vi "Wind Blowing Blizzards.vi"(1 "Valley in":T1[][](array[typedef])) -> (0 "Valley out":T1[][](array[typedef]))   [LabVIEW 2020, in "AoC 2022.lvlib"]
uses:
  AoC 2022.lvlib
  Valley Point.ctl
  Valley Item.ctl
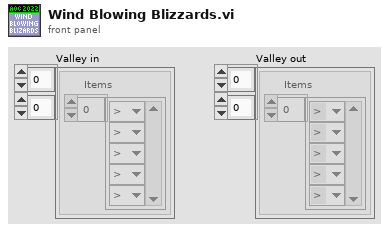
[diagram p1: front panel]
types:
  T1 = typedef "AoC 2022.lvlib/Valley Point.ctl" = cluster{"Items":T2[]}
  T2 = typedef "AoC 2022.lvlib/Valley Item.ctl" = enum16{"#", ".", ">", "<", "^", "v", "E"}
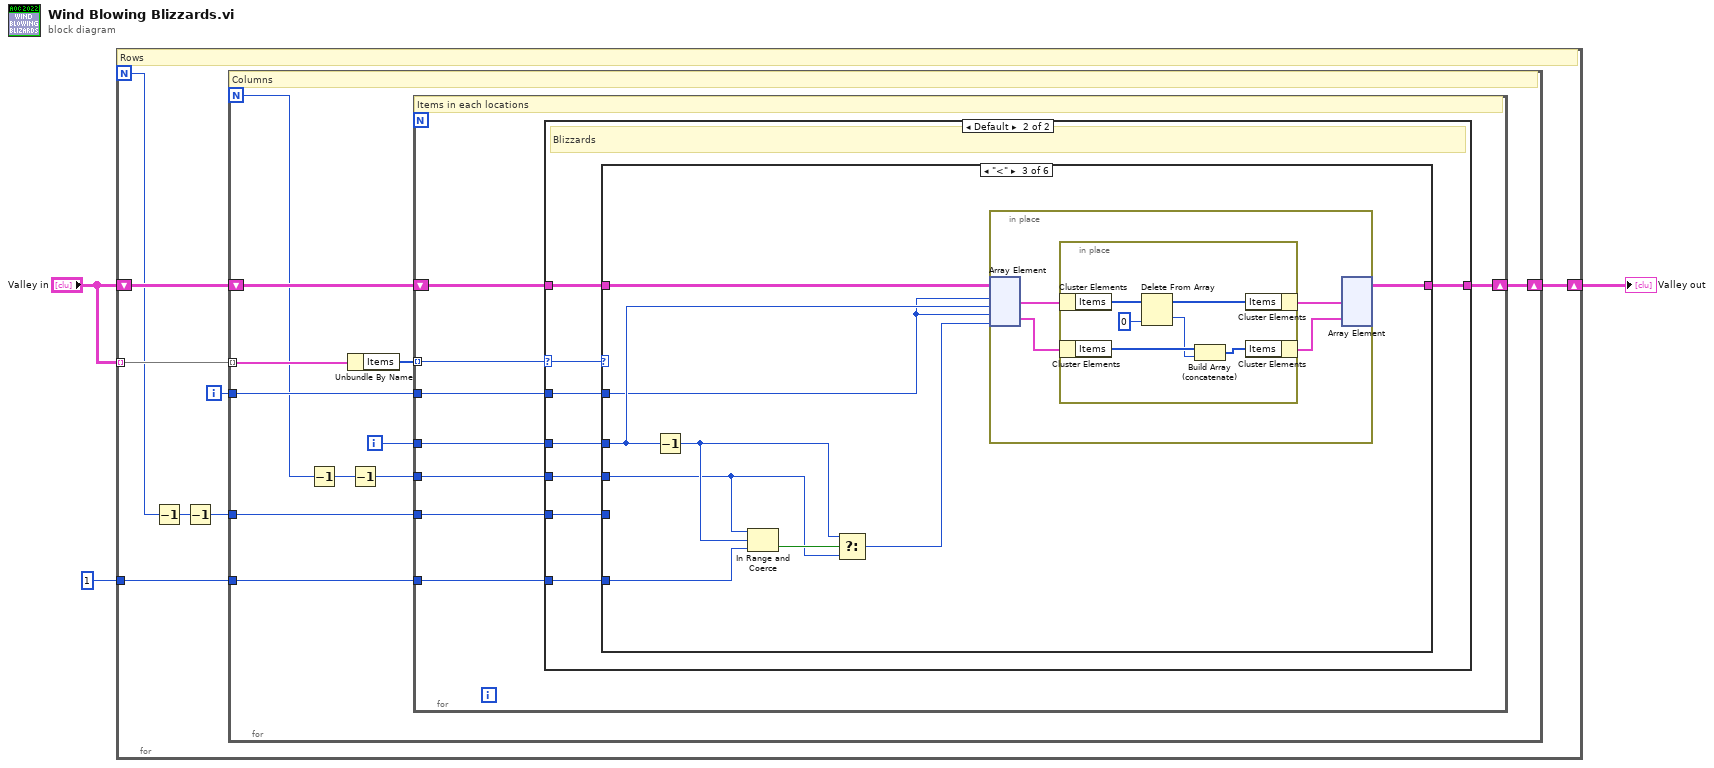
[diagram p0: block diagram]
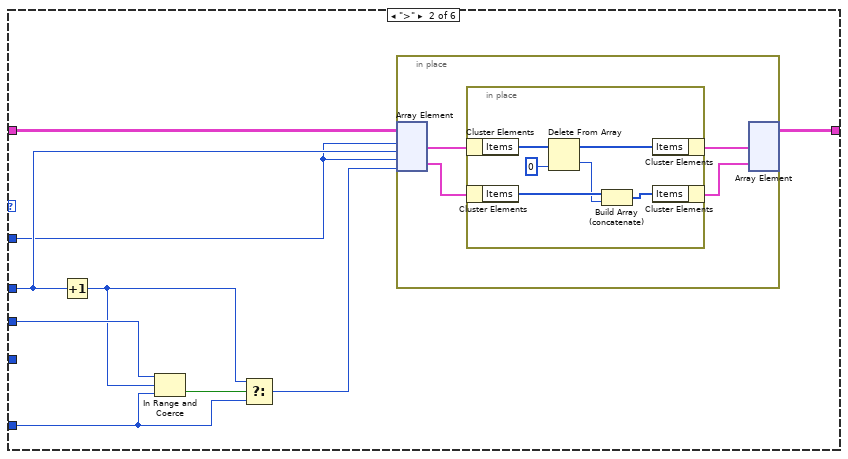
[diagram p4: hidden frame]
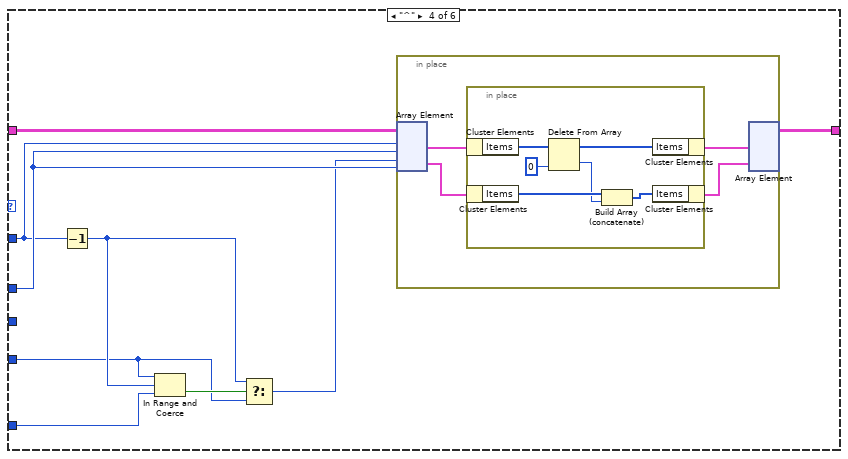
[diagram p5: hidden frame]
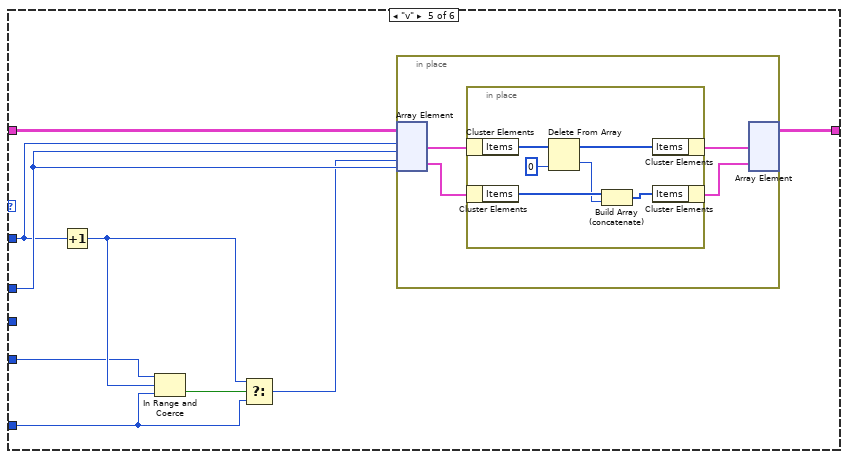
[diagram p6: hidden frame]
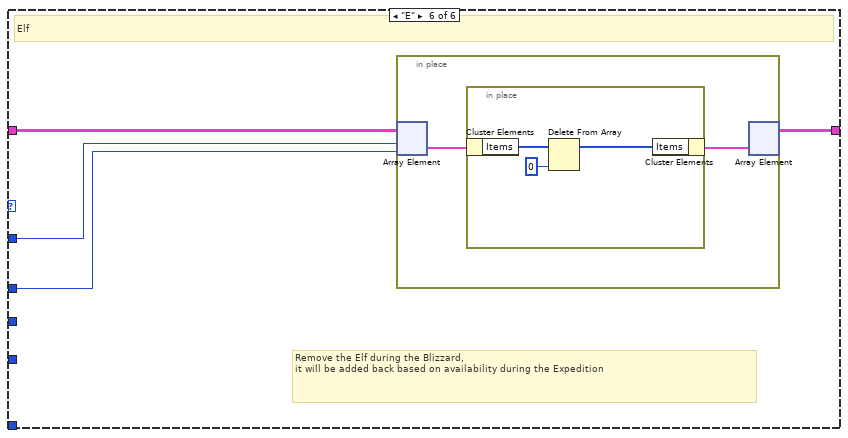
[diagram p7: hidden frame]
diagram:
  n1 = for {
    N -> [w7]
    shift-right: [w10] -> w2
    shift-left: "Valley in" -> [w11]
    tunnel: "Valley in" -> [w9] mode=indexing
    tunnel: 1 -> [w6]
    i -> [w8]
    # "Rows"
    n2 = Decrement(x=w7) -> (x-1=w4:i32)
    n3 = Decrement(x=w4) -> (x-1=w5:i32)
    n4 = for {
      N -> [w15]
      shift-right: [w21] -> w10
      shift-left: w11 -> [w22]
      tunnel: w9 -> [w20] mode=indexing
      tunnel: w8 -> [w18]
      tunnel: w5 -> [w16]
      tunnel: w6 -> [w14]
      i -> [w17]
      # "Columns"
      n5 = Decrement(x=w15) -> (x-1=w12:i32)
      n6 = Unbundle By Name(w20) -> ("Items"=w19:T2[])
      n7 = Decrement(x=w12) -> (x-1=w13:i32)
      n8 = for {
        tunnel: w19 -> [w28] mode=indexing
        shift-right: [w29] -> w21
        shift-left: w22 -> [w30]
        tunnel: w18 -> [w27]
        tunnel: w17 -> [w26]
        tunnel: w16 -> [w25]
        tunnel: w13 -> [w24]
        tunnel: w14 -> [w23]
        # "Items in each locations"
        n9 = case shown="Default" w28 {
          selector: w28 -> [_ w39]
          tunnel: w30 -> [w31 w36]
          tunnel: [w31 w35] -> w29
          tunnel: w27 -> [_ w38]
          tunnel: w26 -> [_ w37]
          tunnel: w25 -> [_ w34]
          tunnel: w24 -> [_ w33]
          tunnel: w23 -> [_ w32]
          frame "#", ".", "E" {
            # "Other Elements"
          }
          frame Default {
            # "Blizzards"
            n10 = case shown="\"<\"" w39 {
              tunnel: w38 -> [_ w41 w62 w80 w100 w117]
              tunnel: w37 -> [_ w42 w63 w82 w102 w118]
              tunnel: w36 -> [w40 w49 w68 w87 w106 w120]
              tunnel: [w40 w48 w67 w86 w105 w119] -> w35
              tunnel: w34 -> [_ _ _ w79 w99 _]
              tunnel: w33 -> [_ w47 w61 _ _ _]
              tunnel: w32 -> [_ w44 w60 w83 w98 _]
              frame "#", "." {
              }
              frame ">" {
                n11 = Increment(x=w42) -> (x+1=w45:i32)
                n12 = In Range and Coerce(upper limit=w47, x=w45, lower limit=w44) -> (In Range?=w46:bool)  [unwired: 1 out]
                n13 = Select(t=w45, s=w46, f=w44) -> (s? t:f=w43:i32)
                n14 = in-place {
                  n15 = in-place-array #1(w49, w41, w42, w41, w43) -> (w53:T1, w51:T1)
                  n16 = in-place {
                    n17 = in-place-cluster #2(w53) -> ("Items"=w59:T2[])
                    n18 = in-place-cluster #3(w51) -> ("Items"=w56:T2[])
                    n19 = Delete From Array(array=w59, index=0) -> (deleted portion=w55:T2, array with subset deleted=w58:T2[])  [unwired: 1 in]
                    n20 = Build Array (concatenate)(w56, w55) -> (w54:T2[])
                    n21 = in-place-cluster #2("Items"=w58) -> (w52:T1)
                    n22 = in-place-cluster #3("Items"=w54) -> (w50:T1)
                  }
                  n23 = in-place-array #1(w52, w50) -> (w48:T1[][])  [unwired: 4 out]
                }
              }
              frame "<" {
                n24 = Decrement(x=w63) -> (x-1=w65:i32)
                n25 = In Range and Coerce(upper limit=w61, x=w65, lower limit=w60) -> (In Range?=w66:bool)  [unwired: 1 out]
                n26 = Select(t=w65, s=w66, f=w61) -> (s? t:f=w64:i32)
                n27 = in-place {
                  n28 = in-place-array #4(w68, w62, w63, w62, w64) -> (w72:T1, w70:T1)
                  n29 = in-place {
                    n30 = in-place-cluster #5(w72) -> ("Items"=w78:T2[])
                    n31 = in-place-cluster #6(w70) -> ("Items"=w75:T2[])
                    n32 = Delete From Array(array=w78, index=0) -> (deleted portion=w74:T2, array with subset deleted=w77:T2[])  [unwired: 1 in]
                    n33 = Build Array (concatenate)(w75, w74) -> (w73:T2[])
                    n34 = in-place-cluster #5("Items"=w77) -> (w71:T1)
                    n35 = in-place-cluster #6("Items"=w73) -> (w69:T1)
                  }
                  n36 = in-place-array #4(w71, w69) -> (w67:T1[][])  [unwired: 4 out]
                }
              }
              frame "^" {
                n37 = Decrement(x=w80) -> (x-1=w84:i32)
                n38 = In Range and Coerce(upper limit=w79, x=w84, lower limit=w83) -> (In Range?=w85:bool)  [unwired: 1 out]
                n39 = Select(t=w84, s=w85, f=w79) -> (s? t:f=w81:i32)
                n40 = in-place {
                  n41 = in-place-array #7(w87, w80, w82, w81, w82) -> (w91:T1, w89:T1)
                  n42 = in-place {
                    n43 = in-place-cluster #8(w91) -> ("Items"=w97:T2[])
                    n44 = in-place-cluster #9(w89) -> ("Items"=w94:T2[])
                    n45 = Delete From Array(array=w97, index=0) -> (deleted portion=w93:T2, array with subset deleted=w96:T2[])  [unwired: 1 in]
                    n46 = Build Array (concatenate)(w94, w93) -> (w92:T2[])
                    n47 = in-place-cluster #8("Items"=w96) -> (w90:T1)
                    n48 = in-place-cluster #9("Items"=w92) -> (w88:T1)
                  }
                  n49 = in-place-array #7(w90, w88) -> (w86:T1[][])  [unwired: 4 out]
                }
              }
              frame "v" {
                n50 = Increment(x=w100) -> (x+1=w103:i32)
                n51 = In Range and Coerce(upper limit=w99, x=w103, lower limit=w98) -> (In Range?=w104:bool)  [unwired: 1 out]
                n52 = Select(t=w103, s=w104, f=w98) -> (s? t:f=w101:i32)
                n53 = in-place {
                  n54 = in-place-array #10(w106, w100, w102, w101, w102) -> (w110:T1, w108:T1)
                  n55 = in-place {
                    n56 = in-place-cluster #11(w110) -> ("Items"=w116:T2[])
                    n57 = in-place-cluster #12(w108) -> ("Items"=w113:T2[])
                    n58 = Delete From Array(array=w116, index=0) -> (deleted portion=w112:T2, array with subset deleted=w115:T2[])  [unwired: 1 in]
                    n59 = Build Array (concatenate)(w113, w112) -> (w111:T2[])
                    n60 = in-place-cluster #11("Items"=w115) -> (w109:T1)
                    n61 = in-place-cluster #12("Items"=w111) -> (w107:T1)
                  }
                  n62 = in-place-array #10(w109, w107) -> (w105:T1[][])  [unwired: 4 out]
                }
              }
              frame "E" {
                # "Remove the Elf during the Blizzard,\nit will be added back based on availability during the Expedition"
                # "Elf"
                n63 = in-place {
                  n64 = in-place-array #13(w120, w117, w118) -> (w122:T1)
                  n65 = in-place {
                    n66 = in-place-cluster #14(w122) -> ("Items"=w125:T2[])
                    n67 = Delete From Array(array=w125, index=0) -> (array with subset deleted=w124:T2[])  [unwired: 1 in, 1 out]
                    n68 = in-place-cluster #14("Items"=w124) -> (w121:T1)
                  }
                  n69 = in-place-array #13(w121) -> (w119:T1[][])  [unwired: 2 out]
                }
              }
            }
          }
        }
      }
    }
  }
  "Valley out" <- w2
